vi "SingleMeas2 - Test.vi"() -> ()   [LabVIEW 2017]
uses:
  AT901 API/Structures/Struct StatisticModeParameter.ctl
  AT901 API/TypeDefinitions/ES_StatisticMode.ctl
  AT901 API/Structures/Struct TransformationPoint.ctl
panel:
  out "Transformation Point":T1={"dVal1"=0.0, "dVal2"=0.0, "dVal3"=0.0, "dStd1"=0.0001, "dStd2"=0.0001, "dStd3"=0.0001, "dCovar12"=0.0, "dCovar13"=0.0, "dCovar23"=0.0}
  in  "Statistic Mode Params":T2
  out "error out":errorcluster
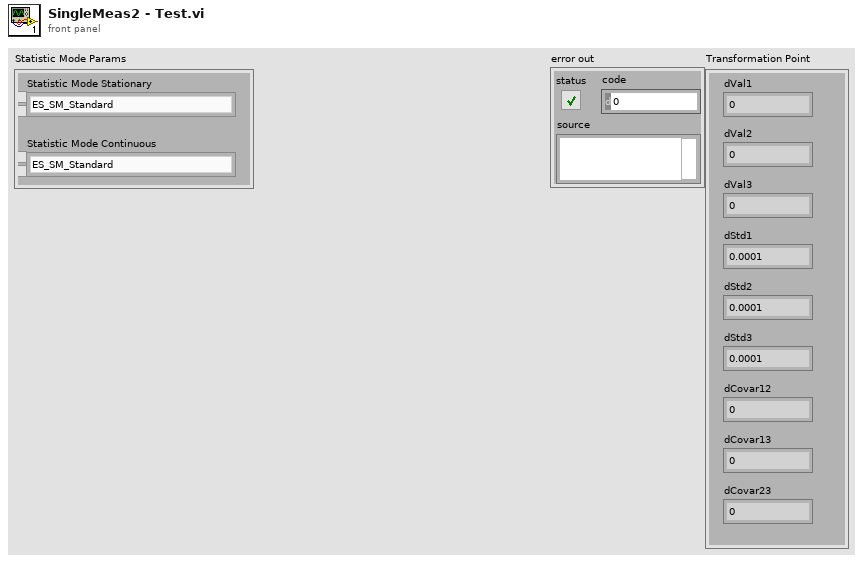
[diagram p1: front panel]
types:
  T1 = typedef "Struct TransformationPoint.ctl" = cluster{"dVal1":dbl, "dVal2":dbl, "dVal3":dbl, "dStd1":dbl, "dStd2":dbl, "dStd3":dbl, "dCovar12":dbl, "dCovar13":dbl, "dCovar23":dbl}
  T2 = typedef "Struct StatisticModeParameter.ctl" = cluster{"Statistic Mode Stationary":T3, "Statistic Mode Continuous":T3}
  T3 = typedef "ES_StatisticMode.ctl" = enum16{"ES_SM_Standard", "ES_SM_Extended"}
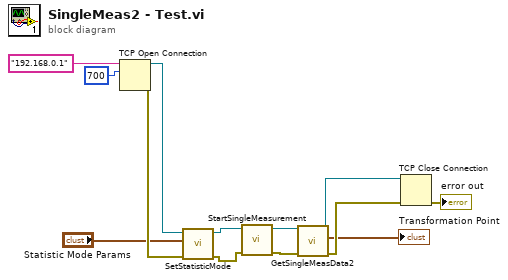
[diagram p0: block diagram]
diagram:
  n1 = TCP Open Connection(address="192.168.0.1", remote port or service name=u16 700) -> (connection ID=w6:refnum<k5>, error out=w5:errorcluster)  [unwired: 3 in]
  n2 = call "SetStatisticMode.vi"("error in (no error)"=w5, "Statistic Mode Params"="Statistic Mode Params", "TCP Network Connection in"=w6) -> ("error out"=w2:errorcluster, "TCP Network Connection out"=w3:refnum<k5>)  [unwired: 5 in, 2 out]
  n3 = call "StartSingleMeasurement.vi"("error in (no error)"=w2, "TCP Network Connection in"=w3) -> ("error out"=w10:errorcluster, "TCP Network Connection out"=w9:refnum<k5>)  [unwired: 7 in, 1 out]
  n4 = call "GetSingleMeasData2.vi"("error in (no error)"=w10, "TCP Network Connection in"=w9) -> ("error out"=w8:errorcluster, "Transformation Point"=→"Transformation Point":T1, "TCP Network Connection out"=w7:refnum<k5>)  [unwired: 6 in, 1 out]
  n5 = TCP Close Connection(connection ID=w7, error in (no error)=w8) -> (error out=→"error out":errorcluster)  [unwired: 1 in, 1 out]
